vi "Vector Expression Test.vi"() -> ()   [LabVIEW 2015]
uses:
  <vilib>/gmath/NI_Gmath.lvlib
panel:
  out "y value":dbl[](array[numeric])=[0.0, 0.5877853083428206, 0.9510565591138008, 0.9510564520671484, 0.5877850280910549, -3.464102066193935e-07, -0.5877855885945158, -0.9510566661603391, -0.9510563450203818, -0.5877847478392194, 6.928204132387453e-07] format="%0.2f"
  in  "expression":string="sin(2*pi*[0:0.1:1])"
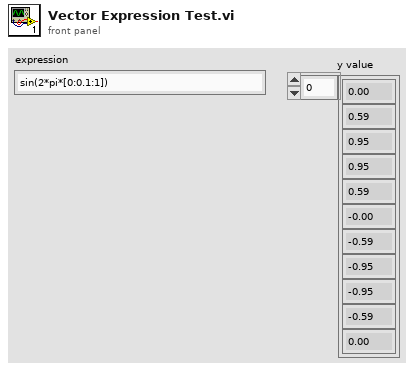
[diagram p1: front panel]
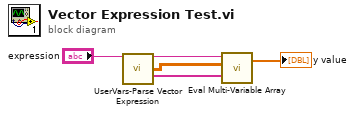
[diagram p0: block diagram]
diagram:
  n1 = call "UserVars-Parse Vector Expression.vi"("Expression In"="expression") -> ("Expression Out"=w4:string, "values"=w3:dbl[][], "variables"=w2:string[])  [unwired: 11 in, 1 out]
  n2 = call <vilib>:"Eval Multi-Variable Array.vi"("Variables"=w2, "X Values"=w3, "formula"=w4) -> ("Y Values"=→"y value":dbl[])  [unwired: 1 in, 1 out]
